vi "Levelmeter_refill_Trap_and_Shield.vi"(0 "Shield Refill":bool, 1 "Stop DAQ":bool, 2 "Trap Refill":bool) -> (4 "Shield control":bool, 5 "Trap control":bool)   [LabVIEW 2019]
uses:
  Global/Global Variables/Data_Display_global.vi
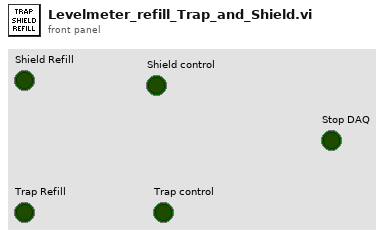
[diagram p1: front panel]
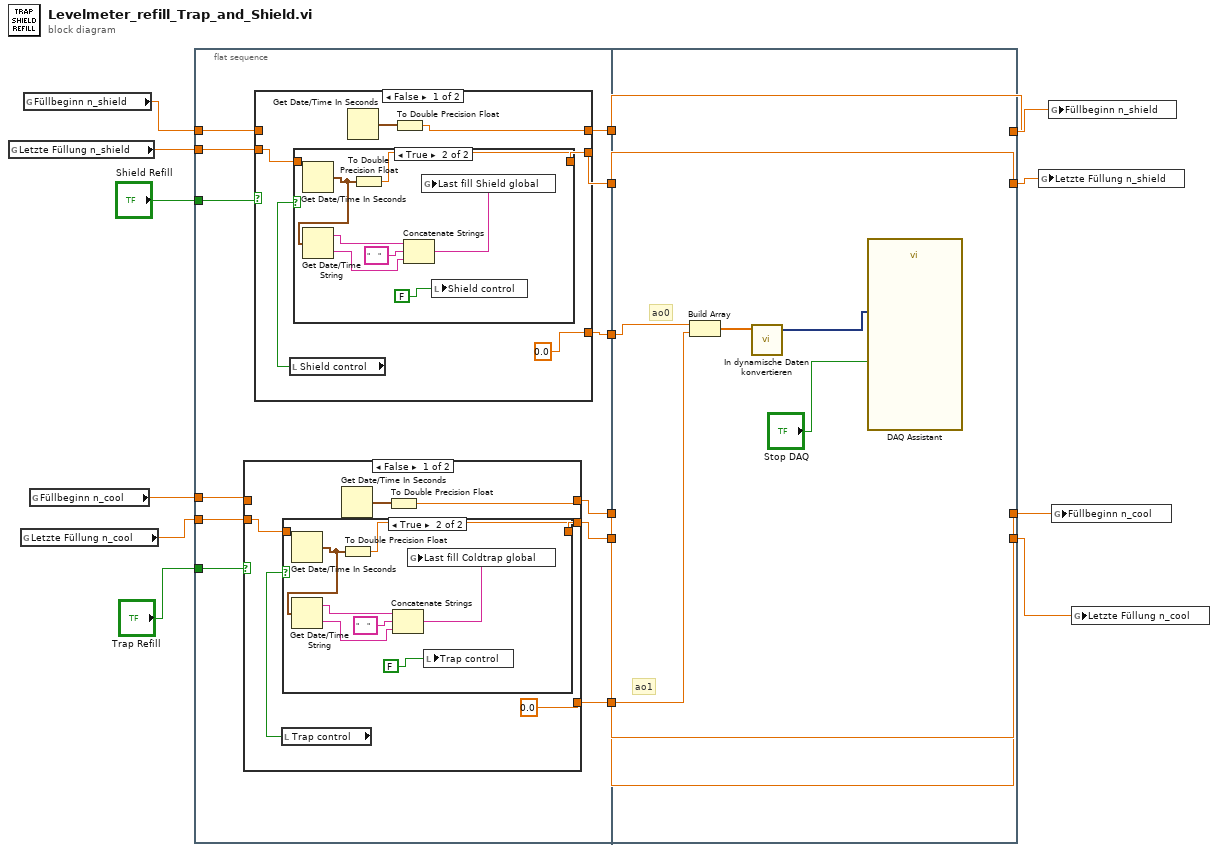
[diagram p0: block diagram]
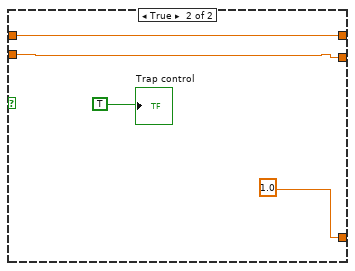
[diagram p3: hidden frame]
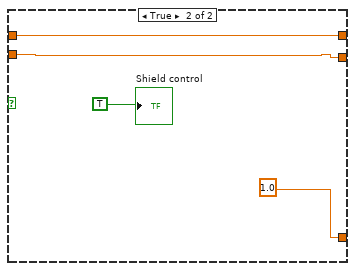
[diagram p5: hidden frame]
diagram:
  n1 = global read "Data_Display_global.vi" "Letzte Füllung n_shield"() -> (w12:dbl)
  n2 = global read "Data_Display_global.vi" "Letzte Füllung n_cool"() -> (w7:dbl)
  n3 = global read "Data_Display_global.vi" "Füllbeginn n_shield"() -> (w13:dbl)
  n4 = global read "Data_Display_global.vi" "Füllbeginn n_cool"() -> (w8:dbl)
  n5 = flat-sequence {
    tunnel: "Shield Refill" -> [w28]
    tunnel: [w27] -> w15
    tunnel: w13 -> [w26]
    tunnel: w12 -> [w25]
    tunnel: [w24] -> w11
    tunnel: [w23] -> w9
    tunnel: w8 -> [w22]
    tunnel: w7 -> [w21]
    tunnel: [w20] -> w6
    tunnel: [w19] -> w4
    tunnel: [w18] -> w2
    tunnel: "Trap Refill" -> [w17]
    tunnel: [w73] -> w14
    tunnel: w15 -> [w73]
    tunnel: [w72] -> w10
    tunnel: w11 -> [w72]
    tunnel: w9 -> [w69]
    tunnel: [w71] -> w5
    tunnel: w6 -> [w71]
    tunnel: [w70] -> w3
    tunnel: w4 -> [w70]
    tunnel: w2 -> [w68]
    frame #0 {
      n6 = case shown="False" w17 {
        tunnel: [w29 w43] -> w20
        tunnel: w22 -> [_ w43]
        tunnel: [w34 w45] -> w19
        tunnel: w21 -> [w32 w45]
        tunnel: [0.0 1.0] -> w18
        frame False {
          n7 = local read "Trap control"() -> (w33:bool)
          n8 = case shown="True" w33 {
            tunnel: [w35 w42] -> w34
            tunnel: w32 -> [w35 _]
            frame False {
            }
            frame True {
              n9 = Get Date/Time In Seconds() -> (seconds since 1Jan1904=w41:timestamp)
              n10 = Get Date/Time String(seconds (now)=w41) -> (date string=w40:string, time string=w38:string)  [unwired: 2 in]
              n11 = To Double Precision Float(number=w41) -> (double precision float=w42:dbl)
              n12 = Concatenate Strings(w40, "    ", w38) -> (w36:string)
              n13 = global write "Data_Display_global.vi" "Last fill Coldtrap global"(w36) -> ()
              n14 = local write "Trap control"(FALSE) -> ()
            }
          }
          n15 = Get Date/Time In Seconds() -> (seconds since 1Jan1904=w30:timestamp)
          n16 = To Double Precision Float(number=w30) -> (double precision float=w29:dbl)
        }
        frame True {
          "Trap control" <- TRUE
        }
      }
      n17 = case shown="False" w28 {
        tunnel: [w47 w61] -> w27
        tunnel: w26 -> [_ w61]
        tunnel: [w51 w63] -> w24
        tunnel: w25 -> [w49 w63]
        tunnel: [0.0 1.0] -> w23
        frame False {
          n18 = local read "Shield control"() -> (w50:bool)
          n19 = case shown="True" w50 {
            tunnel: [w53 w60] -> w51
            tunnel: w49 -> [w53 _]
            frame False {
            }
            frame True {
              n20 = Get Date/Time In Seconds() -> (seconds since 1Jan1904=w59:timestamp)
              n21 = Get Date/Time String(seconds (now)=w59) -> (date string=w58:string, time string=w56:string)  [unwired: 2 in]
              n22 = To Double Precision Float(number=w59) -> (double precision float=w60:dbl)
              n23 = Concatenate Strings(w58, "    ", w56) -> (w54:string)
              n24 = global write "Data_Display_global.vi" "Last fill Shield global"(w54) -> ()
              n25 = local write "Shield control"(FALSE) -> ()
            }
          }
          n26 = Get Date/Time In Seconds() -> (seconds since 1Jan1904=w48:timestamp)
          n27 = To Double Precision Float(number=w48) -> (double precision float=w47:dbl)
        }
        frame True {
          "Shield control" <- TRUE
        }
      }
    }
    frame #1 {
      # "ao1"
      # "ao0"
      n28 = Build Array(w69, w68) -> (w67:dbl[])
      n29 = call "In dynamische Daten konvertieren"("Array"=w67) -> ("Dynamic Data Type"=w66:dynamicdata)  [unwired: 3 in]
      n30 = call "DAQ Assistant"("data"=w66, "stop (T)"="Stop DAQ") -> ()  [unwired: 16 in, 2 out]
    }
  }
  n31 = global write "Data_Display_global.vi" "Letzte Füllung n_shield"(w10) -> ()
  n32 = global write "Data_Display_global.vi" "Füllbeginn n_shield"(w14) -> ()
  n33 = global write "Data_Display_global.vi" "Füllbeginn n_cool"(w5) -> ()
  n34 = global write "Data_Display_global.vi" "Letzte Füllung n_cool"(w3) -> ()
